vi "Reset Manipulator Encoders.vi"(7 "Description":string, 8 "Command Info In":T2, 11 "Reset Parameters":T1) -> (0 "Command Info Out":T2)   [LabVIEW 2020]
doc: "This template is useful for immediate subsystem actions that do not need deadband filtering\n\nBe sure to right-click and select New from Template and save with a new command name."
uses:
  <vilib>/Rock Robotics/WPI/Framework/Command Status Info.ctl
  <vilib>/Rock Robotics/WPI/Framework/Completion Status.ctl
  <vilib>/Rock Robotics/WPI/Framework/Completion Notifier.ctl
  Implementation/manipulator Setpoints.ctl
  Implementation/manipulator Operations.ctl
  Implementation/Typedefs/Teleop Manipulator Commands.ctl
  Implementation/Typedefs/Cube Shooting Presets.ctl
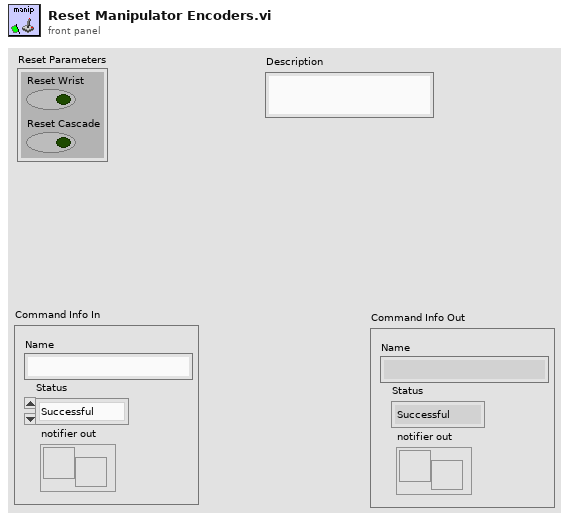
[diagram p1: front panel]
types:
  T1 = cluster{"Reset Wrist":bool, "Reset Cascade":bool}
  T2 = typedef "Command Status Info.ctl" = cluster{"Name":string, "Status":T3, "notifier out":T4}
  T3 = typedef "Completion Status.ctl" = enum16{"Successful", "Aborted", "Incomplete"}
  T4 = typedef "Completion Notifier.ctl" = refnum<notifier>
  T5 = typedef "manipulator Setpoints.ctl" = cluster{"Operation":T6, "Immediate Parameters":cluster{"Wrist Power":dbl, "Cascade Power":dbl}, "Griddy Parameters":cluster{"Griddy Command":T7, "Flip Wrist?":bool}, "Reset Parameters":cluster{"Reset Wrist":bool, "Reset Cascade":bool}, "Shoot Cube Parameters":cluster{"Shot Preset":T8}}
  T6 = typedef "manipulator Operations.ctl" = enum16{"Reserve", "Read Current", "Immediate", "Reset Manipulator", "Grid-dy", "Shoot Cubes"}
  T7 = typedef "Teleop Manipulator Commands.ctl" = enum16{"idle", "intake cone sideways", "intake cone upright", "intake cone feeder", "intake cube feeder", "intake cube", "score low cone", "score low cube", "score mid cone", "score mid cube", "score high cone", "score high cube", "score mid cone up"}
  T8 = typedef "Cube Shooting Presets.ctl" = enum16{"shoot low", "shoot mid", "shoot high"}
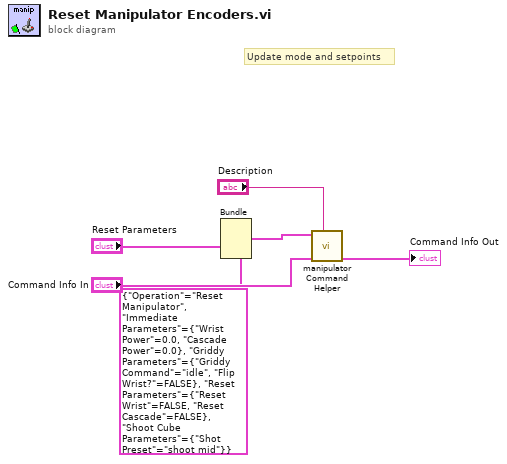
[diagram p0: block diagram]
diagram:
  # "Update mode and setpoints"
  n1 = Bundle(cluster=T5 {"Operation"=enum."Reset Manipulator", "Immediate Parameters"={"Wrist Power"=0.0, "Cascade Power"=0.0}, "Griddy Parameters"={"Griddy Command"=enum."idle", "Flip Wrist?"=FALSE}, "Reset Parameters"={"Reset Wrist"=FALSE, "Reset Cascade"=FALSE}, "Shoot Cube Parameters"={"Shot Preset"=enum."shoot mid"}} ("SubSystem Data"), "Reset Parameters"="Reset Parameters") -> (w2:T5)  [unwired: 4 in]
  n2 = call "manipulator Command Helper.vi"("Description"="Description", "Command Info In"="Command Info In", "SubSystem Data"=w2) -> ("Command Info Out"=→"Command Info Out":T2)  [unwired: 6 in, 2 out]
